vi "电信1801-2018012704-杜兴安-虚拟仪器作业2.vi"() -> ()   [LabVIEW 2020]
panel:
  out "数组 8":dbl[][](array[numeric])
  out "数组 7":dbl[](array[numeric])
  in  "数组 6":dbl[][](array[numeric]) format="%.2f"
  out "所用时间(ms)":dbl
  out "执行次数":dbl
  in  "给定数据":dbl
  in  "b":dbl
  in  "a":dbl
  out "波形图":dbl[][](graph)
  in  "停止":bool
  out "警示灯":bool
  in  "数值 5":dbl
  out "温度计":dbl(slide) scale=0.0..100.0
  out "输出":i32
  in  "输入":ext
  out "数组 5":dbl[](array[numeric])
  out "增加属性后变体":variant
  out "变体":variant
  in  "数组 4":dbl[](array[numeric])
  out "数组 3":cluster{"数值":dbl, "数值 2":dbl, "布尔":bool}[](array[cluster])
  out "数组 2":cluster{"数值":dbl, "数值 2":dbl, "布尔":bool}[](array[cluster])
  in  "姓名":string
  in  "学号":dbl
  out "Cluster 3":cluster{"数值":dbl, "字符串":string, "布尔":bool} caption="簇"
  out "字符串 4":string
  out "布尔 3":bool
  out "数值 4":dbl
  out "字符串 3":string
  out "布尔 2":bool
  out "数组":dbl[][](array[numeric])
  out "数值 3":dbl
  in  "布尔":bool
  in  "字符串 2":string
  in  "数值 2":dbl
  out "Cluster 2":cluster{"数值":dbl, "字符串":string, "布尔":bool} caption="簇"
  in  "字符串":string
  in  "数值":dbl
  out "Cluster":cluster{"数值":dbl, "字符串":string, "布尔":bool} caption="簇"
  # "计算前输入数前所有奇数的和"
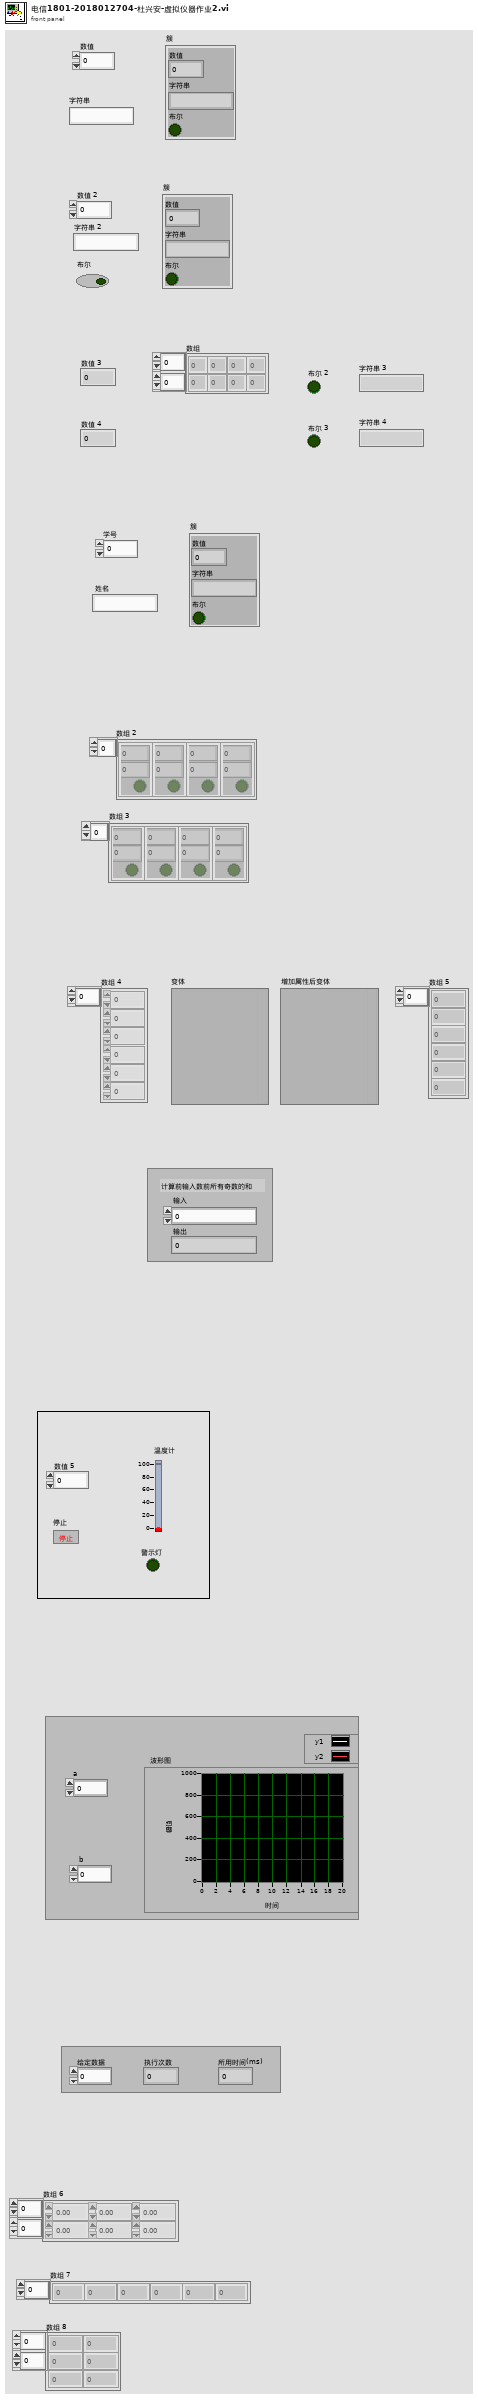
[diagram p1: front panel]
types:
  T1 = cluster{"数值":i32, "数组":dbl[][], "布尔":bool, "字符串":string}
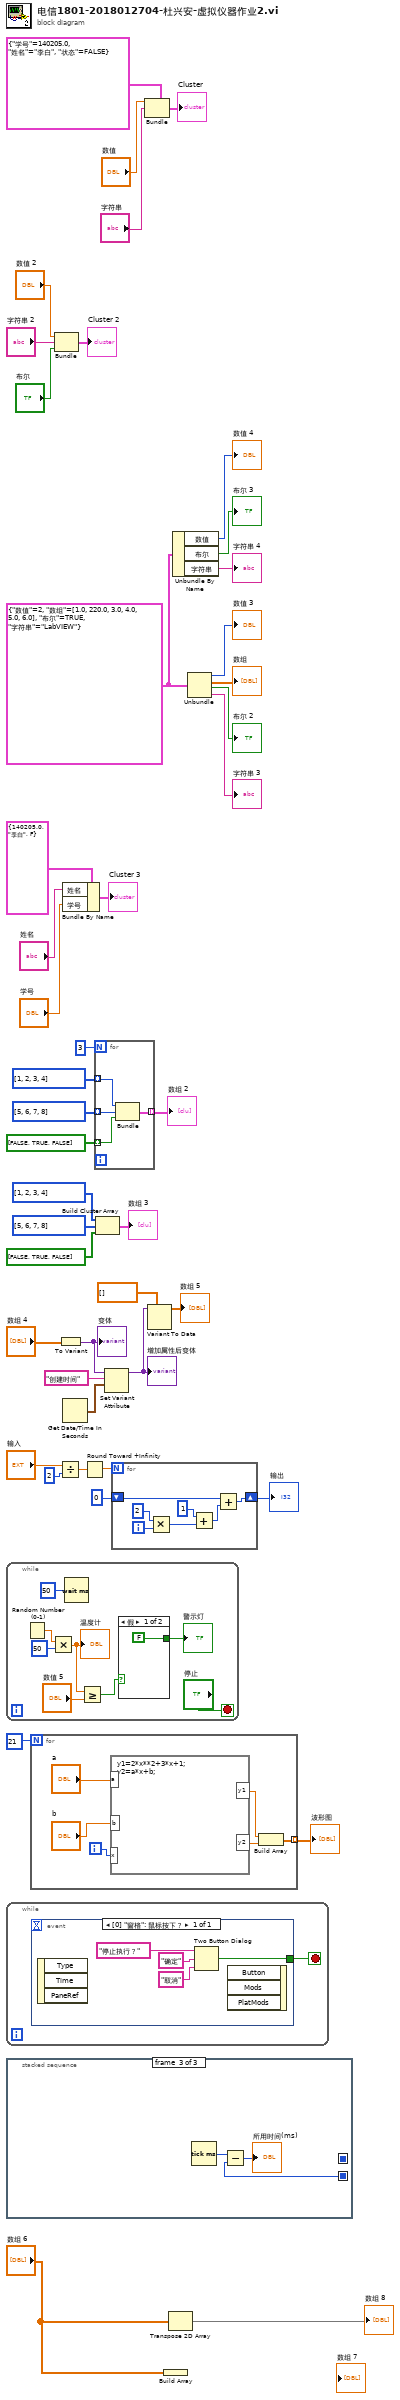
[diagram p0: block diagram]
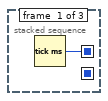
[diagram p2: hidden frame]
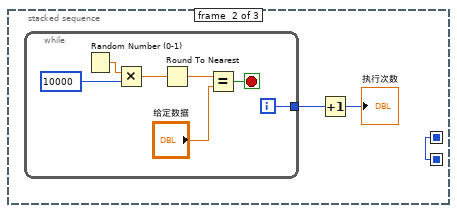
[diagram p3: hidden frame]
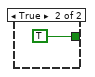
[diagram p4: hidden frame]
diagram:
  w38 = T1 {"数值"=2, "数组"=[[1.0, 220.0, 3.0], [4.0, 5.0, 6.0]], "布尔"=TRUE, "字符串"="LabVIEW"}
  n1 = while {
    stop <- "停止" stop-if-true
    n2 = Random Number (0-1)() -> (number: 0 to 1=w54:dbl)
    n3 = Multiply(x=w54, y=50) -> (x*y=w51:dbl)
    "温度计" <- w51
    n4 = Wait (ms)(milliseconds to wait=50) -> ()  [unwired: 1 out]
    n5 = Greater Or Equal?(x=w51, y="数值 5") -> (x >= y?=w50:bool)
    n6 = case shown="假" w50 {
      tunnel: [FALSE TRUE] -> w47
      frame False {
      }
      frame True {
      }
    }
    "警示灯" <- w47
  }
  n7 = while {
    stop <- w57 stop-if-true
    n8 = event shown="[0] \"窗格\": 鼠标按下？" {
      selector: _ -> [_]
      dyn-events: _ -> [_]
      timeout: _ -> [_]
      tunnel: [w61] -> w57
      event Mouse Down? {
        n9 = event-data() -> ()  [unwired: 1 in, 3 out]
        n10 = Two Button Dialog(message="停止执行？", 1:"取消", 2:"确定") -> (T button?=w61:bool)
        n11 = event-data() -> ()  [unwired: 4 in, 1 out]
      }
    }
  }
  n12 = stacked-sequence {
    seq-local: [w62 _ _] -> [_ w63 _]
    seq-local: [_ w63 _] -> [_ _ w74]
    frame #0 {
      n13 = Tick Count (ms)() -> (millisecond timer value=w62:u32)
    }
    frame #1 {
      n14 = while {
        tunnel: [w67] -> w65
        i -> [w67]
        stop <- w66 stop-if-true
        n15 = Random Number (0-1)() -> (number: 0 to 1=w72:dbl)
        n16 = Multiply(x=w72, y=10000) -> (x*y=w71:dbl)
        n17 = Round To Nearest(number=w71) -> (nearest integer value=w70:dbl)
        n18 = Equal?(x=w70, y="给定数据") -> (x = y?=w66:bool)
      }
      n19 = Increment(x=w65) -> (x+1=→"执行次数":i32)
    }
    frame #2 {
      n20 = Tick Count (ms)() -> (millisecond timer value=w75:u32)
      n21 = Subtract(x=w75, y=w74) -> (x-y=→"所用时间(ms)":u32)
    }
  }
  n22 = for {
    N: 21 -> [_]
    tunnel: [w77] -> w4 mode=indexing
    i -> [w76]
    n23 = formula code="y1=2*x**2+3*x+1;\ny2=a*x+b;"("a"="a", "b"="b", "x"=w76) -> ("y1"=w78:dbl, "y2"=w79:dbl)
    n24 = Build Array(w78, w79) -> (w77:dbl[])
  }
  "波形图" <- w4
  n25 = Bundle("数值 2"="数值 2", "字符串 2"="字符串 2", "布尔"="布尔") -> (→"Cluster 2":cluster{"数值 2":dbl, "字符串 2":string, "布尔":bool})  [unwired: 1 in]
  n26 = Divide(x="输入", y=2) -> (x/y=w5:ext)
  n27 = To Variant(anything="数组 4") -> (Variant=w13:variant)
  "变体" <- w13
  n28 = Bundle By Name(cluster=cluster{"学号":dbl, "姓名":string, "状态":bool} {"学号"=140205.0, "姓名"="李白", "状态"=FALSE}, "姓名"="姓名", "学号"="学号") -> (→"Cluster 3":cluster{"学号":dbl, "姓名":string, "状态":bool})
  n29 = Get Date/Time In Seconds() -> (seconds since 1Jan1904=w15:timestamp)
  n30 = Round Toward +Infinity(x=w5) -> (ceil(x): smallest int >= x=w6:ext)
  n31 = for {
    N: 3 -> [_]
    tunnel: i32[] [1, 2, 3, 4] -> [w85] mode=indexing
    tunnel: i32[] [5, 6, 7, 8] -> [w84] mode=indexing
    tunnel: bool[] [FALSE, TRUE, FALSE] -> [w83] mode=indexing
    tunnel: [w82] -> w18 mode=indexing
    n32 = Bundle(w85, w84, w83) -> (w82:cluster{i32, i32, bool})  [unwired: 1 in]
  }
  "数组 2" <- w18
  n33 = Build Cluster Array(i32[] [1, 2, 3, 4], i32[] [5, 6, 7, 8], bool[] [FALSE, TRUE, FALSE]) -> (→"数组 3":cluster{i32, i32, bool}[])
  n34 = Set Variant Attribute(Variant=w13, name="创建时间", value=w15) -> (Variant out=w14:variant)  [unwired: 1 in, 2 out]
  "增加属性后变体" <- w14
  n35 = for {
    N: w6 -> [_]
    shift-right: [w89] -> w9
    shift-left: 0 -> [w90]
    i -> [w92]
    n36 = Multiply(x=2, y=w92) -> (x*y=w88:i32)
    n37 = Add(x=1, y=w88) -> (x+y=w86:i32)
    n38 = Add(x=w90, y=w86) -> (x+y=w89:i32)
  }
  "输出" <- w9
  n39 = Bundle(cluster=cluster{"学号":dbl, "姓名":string, "状态":bool} {"学号"=140205.0, "姓名"="李白", "状态"=FALSE}, "学号"="数值", "姓名"="字符串") -> (→"Cluster":cluster{"学号":dbl, "姓名":string, "状态":bool})  [unwired: 1 in]
  n40 = Variant To Data(type=dbl[] [], Variant=w14) -> (data=→"数组 5":dbl[])  [unwired: 1 in, 1 out]
  n41 = Build Array("数组 6") -> ()  [unwired: 1 out]
  n42 = Transpose 2D Array(2D array="数组 6") -> (transposed array=→"数组 8":dbl[][])
  n43 = Unbundle By Name(w38) -> ("数值"=→"数值 4":i32, "布尔"=→"布尔 3":bool, "字符串"=→"字符串 4":string)
  n44 = Unbundle(w38) -> ("数值"=→"数值 3":i32, "数组"=→"数组":dbl[][], "布尔"=→"布尔 2":bool, "字符串"=→"字符串 3":string)
